vi "Get Version.vi"(8 "error in (no error)":errorcluster) -> (0 "error out":errorcluster, 2 "Version":T1)   [LabVIEW 2021, in "CIFTemplateNode.lvclass"]
uses:
  CIFTemplateNode.lvclass
  CIFTemplateNode.lvclass/CIFTemplateNode.ctl
  CIFTemplateCommon/Typedef/Version.ctl
  CIFTemplateCommon/CIFTemplateCommon.lvlib
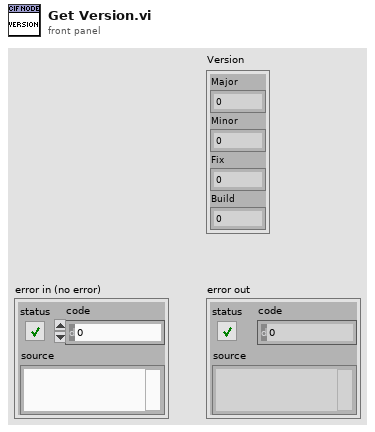
[diagram p1: front panel]
types:
  T1 = typedef "CIFTemplateCommon.lvlib/Version.ctl" = cluster{"Major":i32, "Minor":i32, "Fix":i32, "Build":i32}
  T2 = cluster{"Major":u16, "Minor":u16, "Fix":u16, "Build":u16}
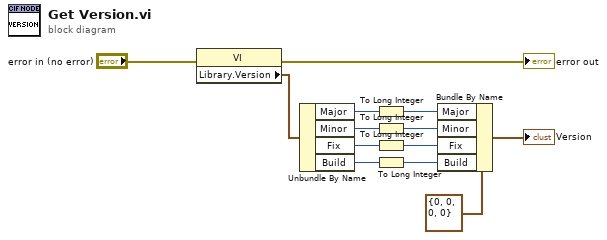
[diagram p0: block diagram]
diagram:
  n1 = property class="VI"(error in="error in (no error)") -> (error out=→"error out":errorcluster, "Library.Version"=w11:T2)  [unwired: 1 in, 1 out]
  n2 = Unbundle By Name(w11) -> ("Major"=w8:u16, "Minor"=w1:u16, "Fix"=w4:u16, "Build"=w5:u16)
  n3 = To Long Integer(number=w8) -> (32bit integer=w7:i32)
  n4 = To Long Integer(number=w1) -> (32bit integer=w2:i32)
  n5 = To Long Integer(number=w4) -> (32bit integer=w3:i32)
  n6 = To Long Integer(number=w5) -> (32bit integer=w6:i32)
  n7 = Bundle By Name(cluster=T1 {"Major"=0, "Minor"=0, "Fix"=0, "Build"=0} ("Version 2"), "Major"=w7, "Minor"=w2, "Fix"=w3, "Build"=w6) -> (→"Version":T1)
